vi "express_node.vi"() -> ()   [LabVIEW 2018]
panel:
  out "Array":dbl[](array[numeric]) caption="배열"
  out "신호":dbl
  out "웨이브폼 그래프":dynamicdata(graph)
  in  "정지 버튼":bool
  out "웨이브폼 차트":dbl(graph)
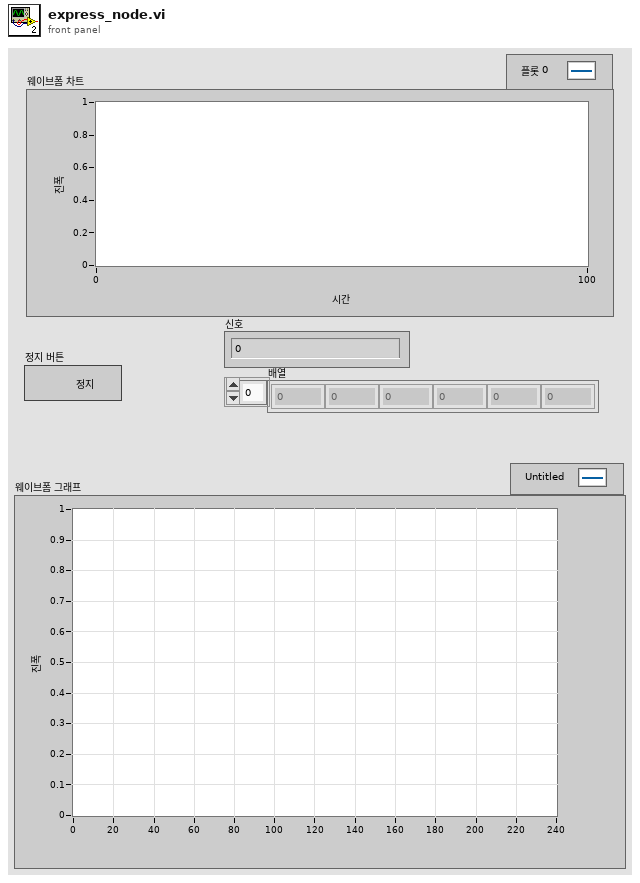
[diagram p1: front panel]
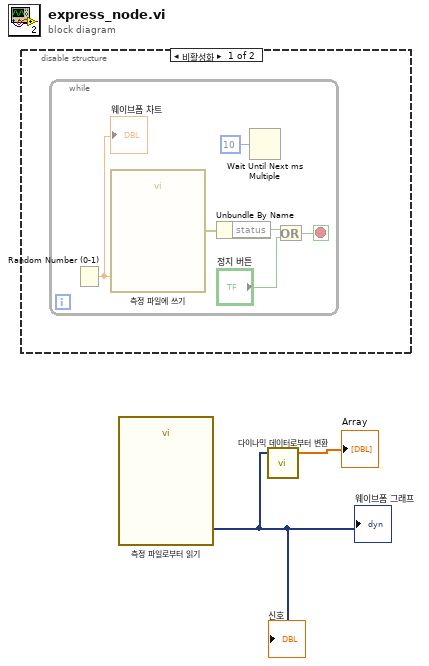
[diagram p0: block diagram]
diagram:
  n1 = disable-structure shown="비활성화" {
    frame Disabled {
      n2 = while {
        stop <- w5 stop-if-true
        n3 = Random Number (0-1)() -> (number: 0 to 1=w8:dbl)
        "웨이브폼 차트" <- w8
        n4 = call "측정 파일에 쓰기"("Signals"=w8) -> ("error out"=w7:errorcluster)  [unwired: 16 in, 2 out]
        n5 = Unbundle By Name(w7) -> ("status"=w6:bool)
        n6 = Wait Until Next ms Multiple(millisecond multiple=u32 10 ("ms 배수")) -> ()  [unwired: 1 out]
        n7 = Or(x=w6, y="정지 버튼") -> (x .or. y?=w5:bool)
      }
    }
    frame Enabled {
    }
  }
  n8 = call "측정 파일로부터 읽기"() -> ("Signals"=w2:dynamicdata)  [unwired: 6 in, 5 out]
  "웨이브폼 그래프" <- w2
  "신호" <- w2
  n9 = call "다이나믹 데이터로부터 변환"("Dynamic Data Type"=w2) -> ("Array"=→"Array":dbl[])  [unwired: 3 in]
